vi "StimFile (G3)-Get Tags.vi"(1 "Path":path) -> (0 "Tags":string[](array[string]))   [LabVIEW 2020]
uses:
  <vilib>/regexp/Match Regular Expression.xnode
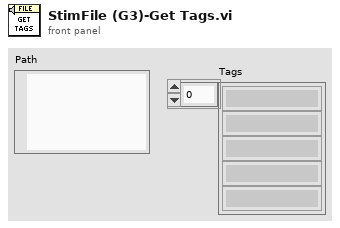
[diagram p1: front panel]
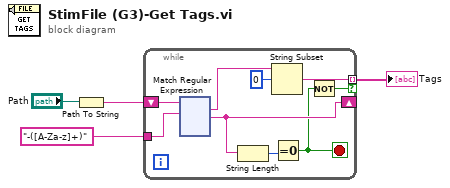
[diagram p0: block diagram]
diagram:
  n1 = Path To String(path="Path") -> (string=w3:string)
  n2 = while {
    tunnel: "-([A-Za-z]+)" ("regular expression") -> [w12]
    tunnel: [w8] -> w1 mode=indexing if=w6
    shift-right: [w10] -> _
    shift-left: w3 -> [w13]
    stop <- w5 stop-if-true
    n3 = xnode "Match Regular Expression"("input string"=w13, "regular expression"=w12) -> ("whole match"=w9:string, "after match"=w10:string)  [unwired: 4 in, 3 out]
    n4 = String Length(string=w10) -> (length=w11:i32)
    n5 = String Subset(string=w9, offset (0)=0) -> (substring=w8:string)  [unwired: 1 in]
    n6 = Equal To 0?(x=w11) -> (x = 0?=w5:bool)
    n7 = Not(x=w5) -> (.not. x?=w6:bool)
  }
  "Tags" <- w1
